vi "1111_#DRIVO.vi"(8 "Refnum in":refnum<k33>, 11 "Dist (m)":dbl) -> (0 "rt fifo out":refnum<k33>)   [LabVIEW 2014]
uses:
  TeleopCmd.ctl
  CmdFlag.ctl
  encoderData.vi
panel:
  in  "Kp":dbl=0.1
  in  "Offset":dbl=0.1
  in  "Thresh":dbl=0.1
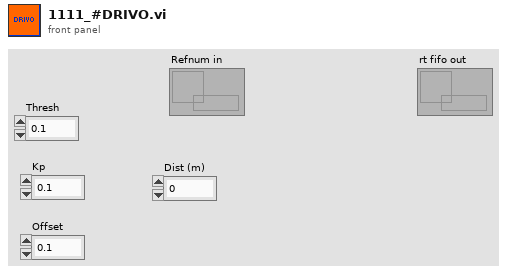
[diagram p1: front panel]
types:
  T1 = typedef "TeleopCmd.ctl" = cluster{"CmdFlag":T2, "throttle":dbl, "turn":dbl, "Override":bool, "Strafe":dbl, "MotorPwrMax":u8, "Time":u32, "ultrasonic override":bool}
  T2 = typedef "CmdFlag.ctl" = enum16{"noop", "logflag", "suspend", "resume"}
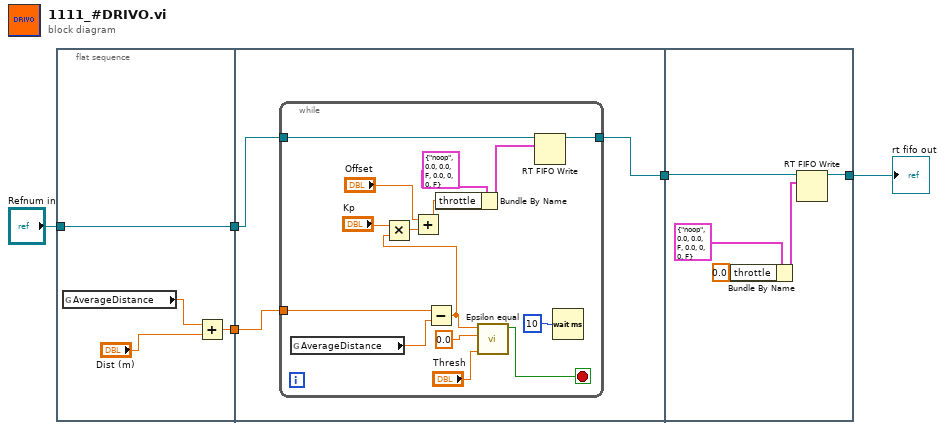
[diagram p0: block diagram]
diagram:
  n1 = flat-sequence {
    tunnel: [w9] -> w5
    tunnel: "Refnum in" -> [w9]
    tunnel: [w6] -> w1
    tunnel: w5 -> [w11]
    tunnel: [w12] -> w4
    tunnel: w1 -> [w10]
    tunnel: [w32] -> w2
    tunnel: w4 -> [w31]
    frame #0 {
      n2 = global read "encoderData.vi" "AverageDistance"() -> (w8:dbl)
      n3 = Add(x=w8, y="Dist (m)") -> (x+y=w6:dbl)
    }
    frame #1 {
      n4 = while {
        tunnel: [w26] -> w12
        tunnel: w11 -> [w25]
        tunnel: w10 -> [w14]
        stop <- w27 stop-if-true
        n5 = global read "encoderData.vi" "AverageDistance"() -> (w13:dbl)
        n6 = Subtract(x=w14, y=w13) -> (x-y=w19:dbl)
        n7 = Multiply(x="Kp", y=w19) -> (x*y=w17:dbl)
        n8 = Add(x="Offset", y=w17) -> (x+y=w18:dbl)
        n9 = Bundle By Name(cluster=T1 {"CmdFlag"=enum."noop", "throttle"=0.0, "turn"=0.0, "Override"=FALSE, "Strafe"=0.0, "MotorPwrMax"=0, "Time"=0, "ultrasonic override"=FALSE} ("Cluster"), "throttle"=w18) -> (w22:T1)
        n10 = call "Epsilon equal.vi"("Epsilon"="Thresh", "Value2"=0.0 ("Epsilon"), "Value1"=w19) -> ("Boolean"=w27:bool)  [unwired: 8 in]
        n11 = RT FIFO Write(0:w25, 1:w22) -> (8:w26:refnum<k33>)  [unwired: 3 in, 3 out]
        n12 = Wait (ms)(milliseconds to wait=u32 10) -> ()  [unwired: 1 out]
      }
    }
    frame #2 {
      n13 = Bundle By Name(cluster=T1 {"CmdFlag"=enum."noop", "throttle"=0.0, "turn"=0.0, "Override"=FALSE, "Strafe"=0.0, "MotorPwrMax"=0, "Time"=0, "ultrasonic override"=FALSE} ("Cluster"), "throttle"=0.0 ("turn")) -> (w29:T1)
      n14 = RT FIFO Write(0:w31, 1:w29) -> (8:w32:refnum<k33>)  [unwired: 3 in, 3 out]
    }
  }
  "rt fifo out" <- w2
